vi "HelloDev.vi"() -> ()   [LabVIEW 2011]
uses:
  API/API DYM.lvlib
panel:
  out "布尔":bool
  in  "退出按钮":bool
  in  "启动按钮":bool
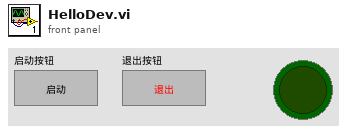
[diagram p1: front panel]
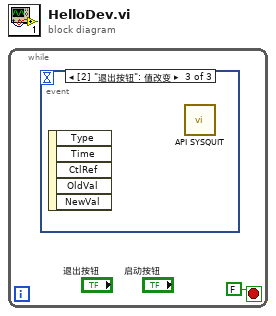
[diagram p0: block diagram]
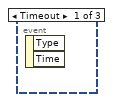
[diagram p2: hidden frame]
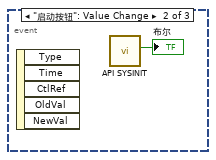
[diagram p3: hidden frame]
diagram:
  n1 = while {
    stop <- FALSE stop-if-true
    n2 = event shown="[2] \"退出按钮\": 值改变" {
      selector: _ -> [_ _ _]
      dyn-events: _ -> [_ _ _]
      timeout: _ -> [_ _ _]
      event Timeout {
        n3 = event-data() -> ()  [unwired: 1 in, 2 out]
      }
      event "启动按钮": Value Change {
        n4 = event-data() -> ()  [unwired: 1 in, 5 out]
        n5 = call "API SYSINIT.vi"() -> ("SYSINIT return value"=→"布尔":bool)  [unwired: 11 in]
      }
      event "退出按钮": Value Change {
        n6 = event-data() -> ()  [unwired: 1 in, 5 out]
        n7 = call "API SYSQUIT.vi"() -> ()  [unwired: 12 in]
      }
    }
  }
